vi "Request Data JSON.vi"(8 "error in (no error)":errorcluster, 11 "CreateSceneCollection in":refnum<class "CreateSceneCollection.lvclass">) -> (0 "error out":errorcluster, 2 "Request Data JSON":string, 3 "CreateSceneCollection out":refnum<class "CreateSceneCollection.lvclass">)   [LabVIEW 2020, in "obs-websocket.lvlib" / "CreateSceneCollection.lvclass"]
uses:
  CreateSceneCollection.lvclass
  CreateSceneCollection.lvclass/CreateSceneCollection.ctl
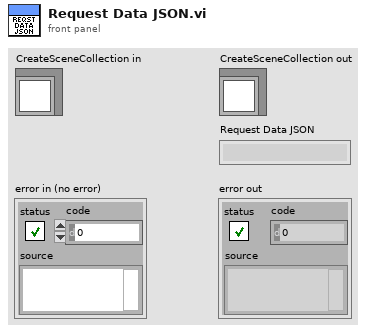
[diagram p1: front panel]
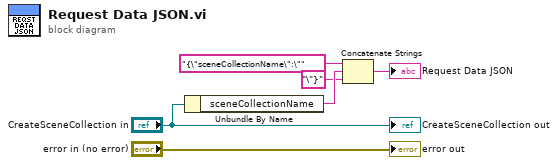
[diagram p0: block diagram]
diagram:
  n1 = Unbundle By Name("CreateSceneCollection in") -> ("sceneCollectionName"=w4:string)
  n2 = Concatenate Strings("{\"sceneCollectionName\":\"" ("string"), w4, "\"}" ("string")) -> (→"Request Data JSON":string)
  "error out" <- "error in (no error)"
  "CreateSceneCollection out" <- "CreateSceneCollection in"
